vi "WPI_ADI_IMU_Reset.vi"(8 "error in":errorcluster, 10 "Reset? (T)":bool=TRUE, 11 "ADI IMU Interrupt DevRef":T1 {"SimpleGyroDevRef"."Sample Rate" min=0.25 max=100.0 step=0.25}) -> (0 "error out":errorcluster, 3 "ADI IMU DevRef":T2 {"Sample Rate" min=0.25 max=100.0 step=0.25})   [LabVIEW 2015, in "FRC ADI MXP IMU.lvlib"]
doc: "Resets the accumulated angles to zero in software. This VI does NOT electrically reset the ADI MXP IMU or reset the calibration."
uses:
  FRC ADI MXP IMU.lvlib
  WPI_AnalogDevicesIMUDevRef.ctl
  <vilib>/Rock Robotics/SystemInterfaces/spilib/spi_bus.ctl
  WPI_AnalogDevicesIMUInterruptDevRef.ctl
  <vilib>/Rock Robotics/WPI/Interrupt/WPI_InterruptRef.ctl
  <vilib>/Rock Robotics/SystemInterfaces/Interrupt/FPGA_InterruptIndex.ctl
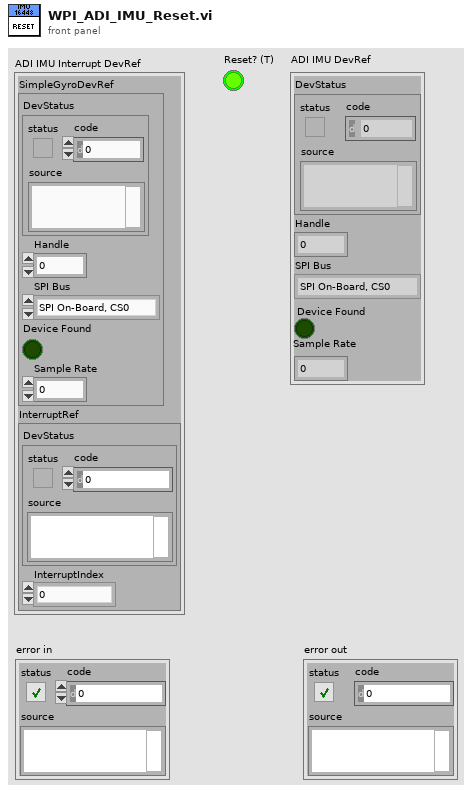
[diagram p1: front panel]
types:
  T1 = typedef "FRC ADI MXP IMU.lvlib/WPI_AnalogDevicesIMUInterruptDevRef.ctl" = cluster{"SimpleGyroDevRef":T2, "InterruptRef":T4}
  T2 = typedef "FRC ADI MXP IMU.lvlib/WPI_AnalogDevicesIMUDevRef.ctl" = cluster{"DevStatus":errorcluster, "Handle":i32, "SPI Bus":T3, "Device Found":bool, "Sample Rate":dbl}
  T3 = typedef "spi_bus.ctl" = enum16{"SPI On-Board, CS0", "SPI On-Board, CS1", "SPI On-Board, CS2", "SPI On-Board, CS3", "SPI MXP", "Invalid"}
  T4 = typedef "WPI_InterruptRef.ctl" = cluster{"DevStatus":errorcluster, "InterruptIndex":T5}
  T5 = typedef "FPGA_InterruptIndex.ctl" = enum8{"0", "1", "2", "3", "4", "5", "6", "7", "Invalid"}
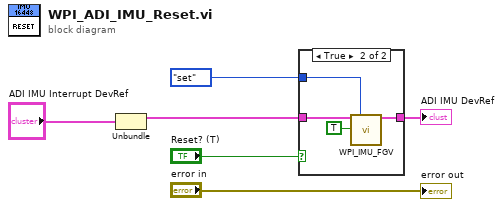
[diagram p0: block diagram]
diagram:
  n1 = Unbundle("ADI IMU Interrupt DevRef") -> ("SimpleGyroDevRef"=w2:T2)  [unwired: 1 out]
  n2 = case shown="True" "Reset? (T)" {
    tunnel: [w7 w11] -> w6
    tunnel: w2 -> [w7 w10]
    tunnel: enum16{"set", "get"}."set" ("Operation") -> [_ w9]
    frame False {
    }
    frame True {
      n3 = call "WPI_IMU_FGV.vi"("SimpleGyroDevRef"=w10, "Operation"=w9, "Reset"=TRUE) -> ("SimpleGyroDevRef"=w11:T2)  [unwired: 8 in, 4 out]
    }
  }
  "ADI IMU DevRef" <- w6
  "error out" <- "error in"
